vi "Init.vi"(8 "error in (no error)":errorcluster, 11 "RHS_2D_Numeric":refnum<class "NI_RHS_2D_Numeric.lvclass">) -> (0 "error out":errorcluster, 3 "initialized RHS_2D_Numeric":refnum<class "NI_RHS_2D_Numeric.lvclass">)   [LabVIEW 2020, in "NI_PDE.lvlib" / "NI_RHS_2D_Numeric.lvclass"]
uses:
  <vilib>/gmath/pde.llb/RHSClass/RHS_2D_Numeric/NI_RHS_2D_Numeric.lvclass
  <vilib>/gmath/pde.llb/RHSClass/Class Type.ctl
  <vilib>/gmath/pde.llb/RHSClass/RHS_2D_Numeric/NI_RHS_2D_Numeric.lvclass/NI_RHS_2D_Numeric.ctl
  <vilib>/gmath/pde.llb/RHSClass/NI_RHS.lvclass
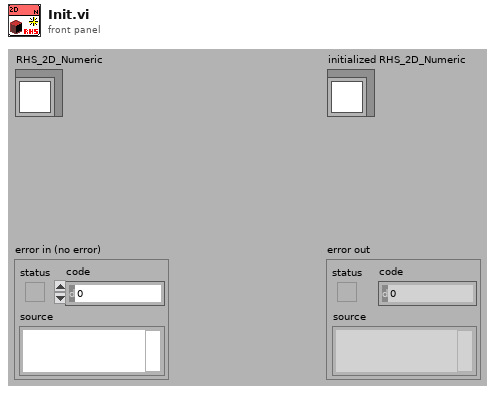
[diagram p1: front panel]
types:
  T1 = typedef "NI_PDE.lvlib/NI_RHS.lvclass/Class Type.ctl" = i32
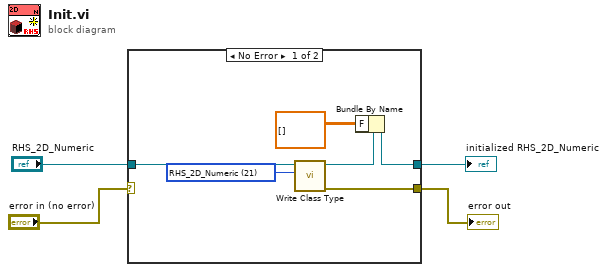
[diagram p0: block diagram]
diagram:
  n1 = case shown="No Error" "error in (no error)" {
    selector: "error in (no error)" -> [_ w11]
    tunnel: [w7 w12] -> w4
    tunnel: [w6 w11] -> w3
    tunnel: "RHS_2D_Numeric" -> [w9 w12]
    frame No Error {
      w10 = T1 21 items=["RHS"=0, "RHS_2D"=20, "RHS_2D_Numeric"=21, "RHS_2D_VIRef"=22, "RHS_3D"=30, "RHS_3D_Numeric"=31, "RHS_3D_VIRef"=32] ("RHS class type")
      n2 = call-dynamic "Write Class Type.vi"("RHS class type"=w10, "RHS.lvclass in"=w9) -> ("error out"=w6:errorcluster, "RHS.lvclass out"=w8:refnum<class "NI_RHS_2D_Numeric.lvclass">)  [unwired: 1 in, 7 out]
      n3 = Bundle By Name(cluster=w8, "F"=dbl[][] []) -> (w7:refnum<class "NI_RHS_2D_Numeric.lvclass">)
    }
    frame Error {
    }
  }
  "initialized RHS_2D_Numeric" <- w4
  "error out" <- w3
